vi "FL_Last_N_Samples_2D_array_of_strings.vi"(1 "BufferLengthSamples":u32=10, 2 "Input Array of strings":string[][](array[string])) -> (0 "Output Array of strings":string[][](array[string]))   [LabVIEW 2018, in "Tracker.lvlib"]
uses:
  Tracker.lvlib
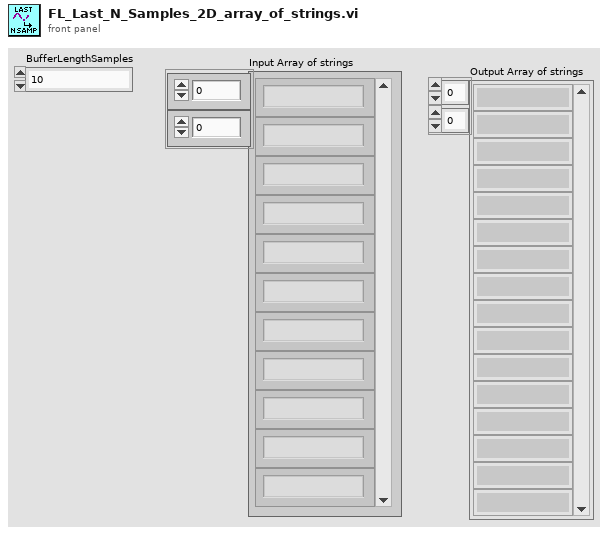
[diagram p1: front panel]
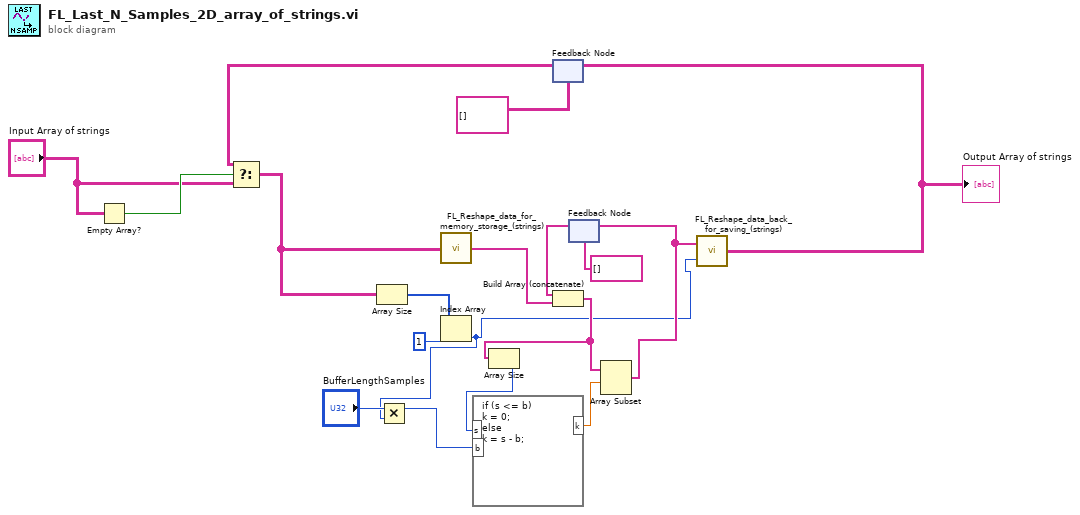
[diagram p0: block diagram]
diagram:
  n1 = Empty Array?(array="Input Array of strings") -> (empty?=w5:bool)
  n2 = feedback #1(string[][] []) -> (w3:string[][])
  n3 = Select(t=w3, s=w5, f="Input Array of strings") -> (s? t:f=w6:string[][])
  n4 = Array Size(array=w6) -> (size(s)=w13:i32[])
  n5 = call "FL_Reshape_data_for_memory_storage_(strings).vi"("DEC string input"=w6) -> ("DEC string output"=w10:string[])
  n6 = Index Array(array=w13, index=1) -> (element=w7:i32)
  n7 = Multiply(x="BufferLengthSamples", y=w7) -> (x*y=w11:u32)
  n8 = feedback #2(string[] []) -> (w18:string[])
  n9 = Build Array (concatenate)(w18, w10) -> (w17:string[])
  n10 = Array Size(array=w17) -> (size(s)=w16:i32)
  n11 = formula code="if (s <= b)\nk = 0;\nelse\nk = s - b;"("s"=w16, "b"=w11) -> ("k"=w15:dbl)
  n12 = Array Subset(array=w17, index=w15) -> (w8:string[])  [unwired: 1 in]
  n13 = feedback-in #2(w8) -> ()
  n14 = call "FL_Reshape_data_back_for_saving_(strings).vi"("Read frame size"=w7, "DEC string input"=w8) -> ("DEC string output"=w1:string[][])
  "Output Array of strings" <- w1
  n15 = feedback-in #1(w1) -> ()
